vi "Modbus RT Driver VI.vi"(6 "Device Clock":string, 9 "Device Inputs FIFO":refnum<k33>, 10 "Device Outputs FIFO":refnum<k33>, 11 "Device Reference":T11 format="%.0x") -> ()   [LabVIEW 2014, in "Modbus Engine.lvlib"]
uses:
  Modbus Engine.lvlib
  <vilib>/NI Veristand/Custom Device API/Custom Device Item Ref.ctl
  XML Deserializer/XML VIs/API/Controls/Modbus_Items.ctl
  XML Deserializer/XML VIs/API/Controls/Modbus_Item_Type.ctl
  Shared/FIFO Indexes.ctl
  <vilib>/NI Veristand/Custom Device API/Custom Device Channel Type.ctl
  XML Deserializer/XML VIs/API/Controls/Modbus_General_Settings.ctl
  XML Deserializer/XML VIs/API/Controls/Modbus_Communication_Type.ctl
  XML Deserializer/XML VIs/API/Controls/Modbus_Type.ctl
  XML Deserializer/XML VIs/API/Controls/Modbus_Serial_Settings_Flow_Control.ctl
  XML Deserializer/XML VIs/API/Controls/Modbus_Serial_Settings_Parity.ctl
  XML Deserializer/XML VIs/API/Controls/Modbus_Serial_Settings_Serial_Type.ctl
  <vilib>/NI Veristand/Custom Device API/Message Response (String).ctl
  <vilib>/NI Veristand/Custom Device API/Message Response (Byte Array).ctl
  <vilib>/NI Veristand/Custom Device Tools/Custom Device Utility Library/RT Debug String Color Spec.ctl
  <vilib>/NI Veristand/Custom Device API/Get Item Property (Variant).vi
  Glyphs/Modbus Property Names.vi
  <vilib>/NI Veristand/Custom Device API/Custom Device API.lvlib
  <vilib>/NI Veristand/Custom Device Tools/Custom Device Utility Library/Custom Device Utility Library.lvlib
  Shared/Modbus Shared.lvlib
  <vilib>/NI_Real-Time Target Support.lvlib
panel:
  in  "Inputs RT-FIFO":dbl[](array[numeric])=[0.0, 0.0, 0.0, 0.0, 0.0, 0.0, 0.0, 0.0, 0.0, 0.0, 0.0, 0.0, 0.0, 0.0, 0.0, 0.0, 0.0, 0.0, 0.0, 0.0, 0.0, 0.0, 0.0, 0.0, 0.0, 0.0, 0.0, 0.0, 0.0, 0.0]
  out "Outputs RT-FIFO":dbl[](array[numeric])
  out "DEBUG error IO":errorcluster
  in  "DEBUG stop":bool
  out "DEBUG General Settings":T1 {"Communication_Type" items=["TCP", "Serial"]; "Modbus_Type" items=["Master", "Slave"]; "Serial Settings"."Serial_Settings_Flow_Control" items=["None", "XONXOFF", "RTSCTS", "XONXOFFANDRTSCTS", "DTRDSR", "XONXOFFANDDTRDSR"]; "Serial Settings"."Serial_Settings_Parity" items=["None", "Odd", "Even"]; "Serial Settings"."Serial_Settings_Serial_Type" items=["RTU", "ASCII"]}
  out "DEBUG RT-FIFOs Indexes":T7[](array[typedef])
  out "DEBUG Modbus Items":T9[](array[typedef])
  in  "Initialization Status Notifier":refnum<notifier>
  in  "Status Notifier":refnum<notifier>
  # "Custom Device Template\nv1.0"
  # "Use this template as a starting point for creating a custom device code module. The input controls shown here are specially named controls that the system will use to provide the device loop with data. The controls are not required for the device loop to run. For instance, if the device doesn't produce any output data, then you don't need the Device Outputs FIFO control. If you do use these controls, however, they need to have these exact names to be functional."
  # "The optional status notifier element is used to notify the RT engine of the last state of the custom device, and to indicate the device has completed execution. If this control is not used, a default No Error value is returned to the system when the device finishes execution.\n\nNote: This error state is not checked until the system shuts down. Use an output status channel to send more immediate status values to the system."
  # "This optional input can be used to send the VeriStand Engine the final status of the custom device initalization process. If this control exists on the custom device front panel, the VeriStand Engine will wait for a status update before starting up. If the custom device reports an error, that will abort the execution of the current configuration in the VeriStand Engine.\n\nThis control can be deleted if the custom device does not need to send the initialization status update."
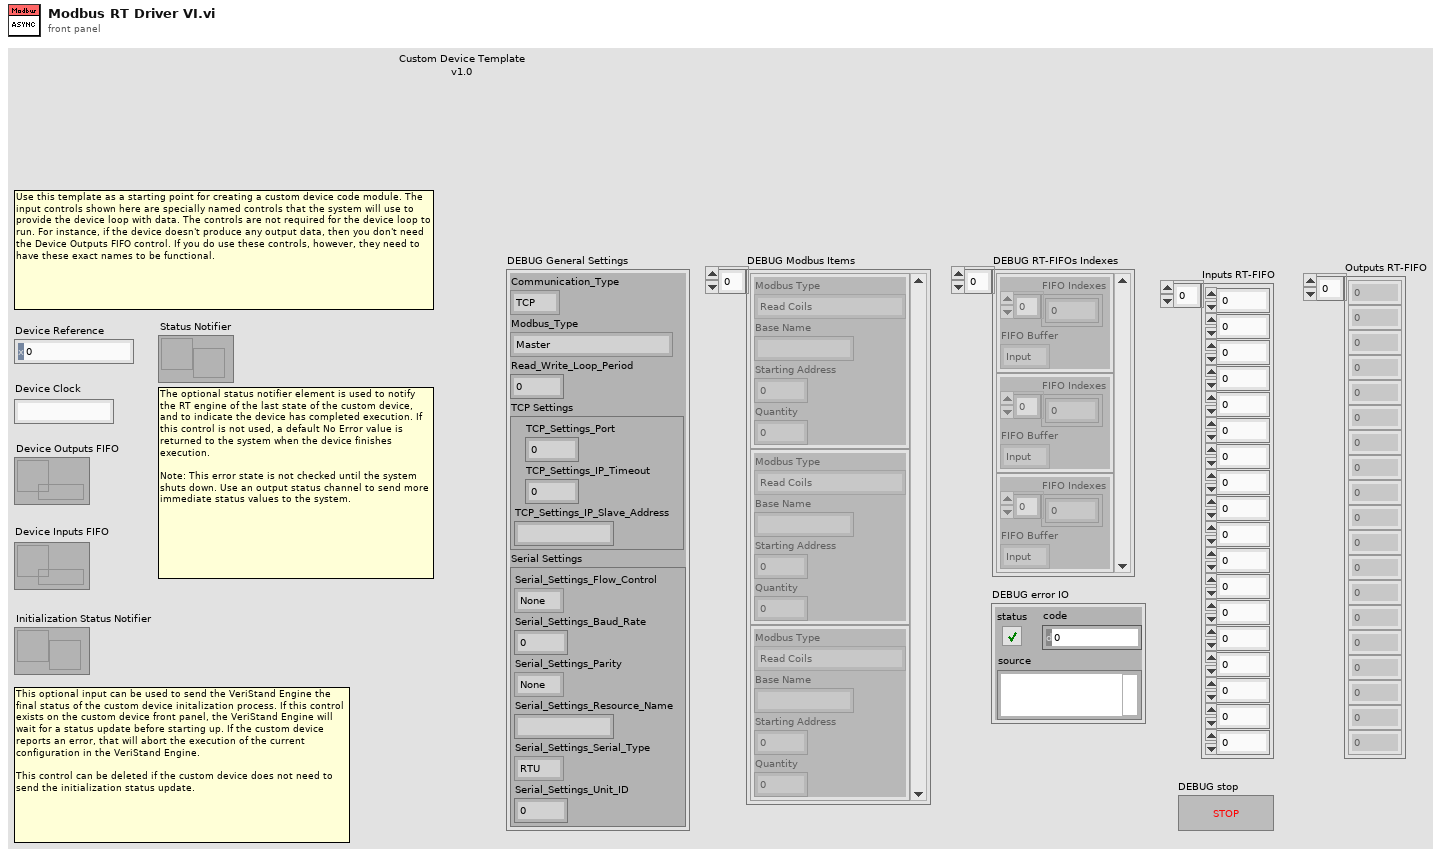
[diagram p1: front panel]
types:
  T1 = typedef "Modbus Shared.lvlib/Modbus_General_Settings.ctl" = cluster{"Communication_Type":T2, "Modbus_Type":T3, "Read_Write_Loop_Period":i64, "TCP Settings":cluster{"TCP_Settings_Port":u16, "TCP_Settings_IP_Timeout":u32, "TCP_Settings_IP_Slave_Address":string}, "Serial Settings":cluster{"Serial_Settings_Flow_Control":T4, "Serial_Settings_Baud_Rate":u32, "Serial_Settings_Parity":T5, "Serial_Settings_Resource_Name":string, "Serial_Settings_Serial_Type":T6, "Serial_Settings_Unit_ID":u8}}
  T2 = typedef "Modbus Shared.lvlib/Modbus_Communication_Type.ctl" = i32
  T3 = typedef "Modbus Shared.lvlib/Modbus_Type.ctl" = i32
  T4 = typedef "Modbus Shared.lvlib/Modbus_Serial_Settings_Flow_Control.ctl" = i32
  T5 = typedef "Modbus Shared.lvlib/Modbus_Serial_Settings_Parity.ctl" = i32
  T6 = typedef "Modbus Shared.lvlib/Modbus_Serial_Settings_Serial_Type.ctl" = i32
  T7 = typedef "Modbus Shared.lvlib/FIFO Indexes.ctl" = cluster{"FIFO Indexes":i32[], "FIFO Buffer":T8}
  T8 = typedef "Custom Device API.lvlib/Custom Device Channel Type.ctl" = enum16{"Input", "Output"}
  T9 = typedef "Modbus Shared.lvlib/Modbus_Items.ctl" = cluster{"Modbus Type":T10, "Base Name":string, "Starting Address":u16, "Quantity":u16}
  T10 = typedef "Modbus Shared.lvlib/Modbus_Item_Type.ctl" = enum16{"Read Coils", "Read Discrete Inputs", "Read Holding Registers", "Read Input Registers", "Write Multiple Coils", "Write Multiple Holding Registers", "Write Single Coil", "Write Single Holding Register", "Write Multiple Discrete Inputs", "Write Multiple Input Registers"}
  T11 = typedef "Custom Device API.lvlib/Custom Device Item Ref.ctl" = u64
  T12 = typedef "Custom Device API.lvlib/Custom Device Item Info.ctl" = cluster{"Name":string, "Is Channel":bool, "GUID":string, "Is Waveform":bool}
  T13 = typedef "Custom Device API.lvlib/Custom Device Engine Event Ref.ctl" = refnum<event-registration>
  T14 = cluster{"TCP_Settings_Port":u16, "TCP_Settings_IP_Timeout":u32, "TCP_Settings_IP_Slave_Address":string}
  T15 = cluster{"Serial_Settings_Flow_Control":T4, "Serial_Settings_Baud_Rate":u32, "Serial_Settings_Parity":T5, "Serial_Settings_Resource_Name":string, "Serial_Settings_Serial_Type":T6, "Serial_Settings_Unit_ID":i8}
  T16 = typedef "Custom Device API.lvlib/Message Response (String).ctl" = cluster{"Response":string, "Error":errorcluster}
  T17 = typedef "Custom Device API.lvlib/Message Response (Byte Array).ctl" = cluster{"Response":u8[], "Error":errorcluster}
  T18 = typedef "Custom Device Utility Library.lvlib/RT Debug String Color Spec.ctl" = u16
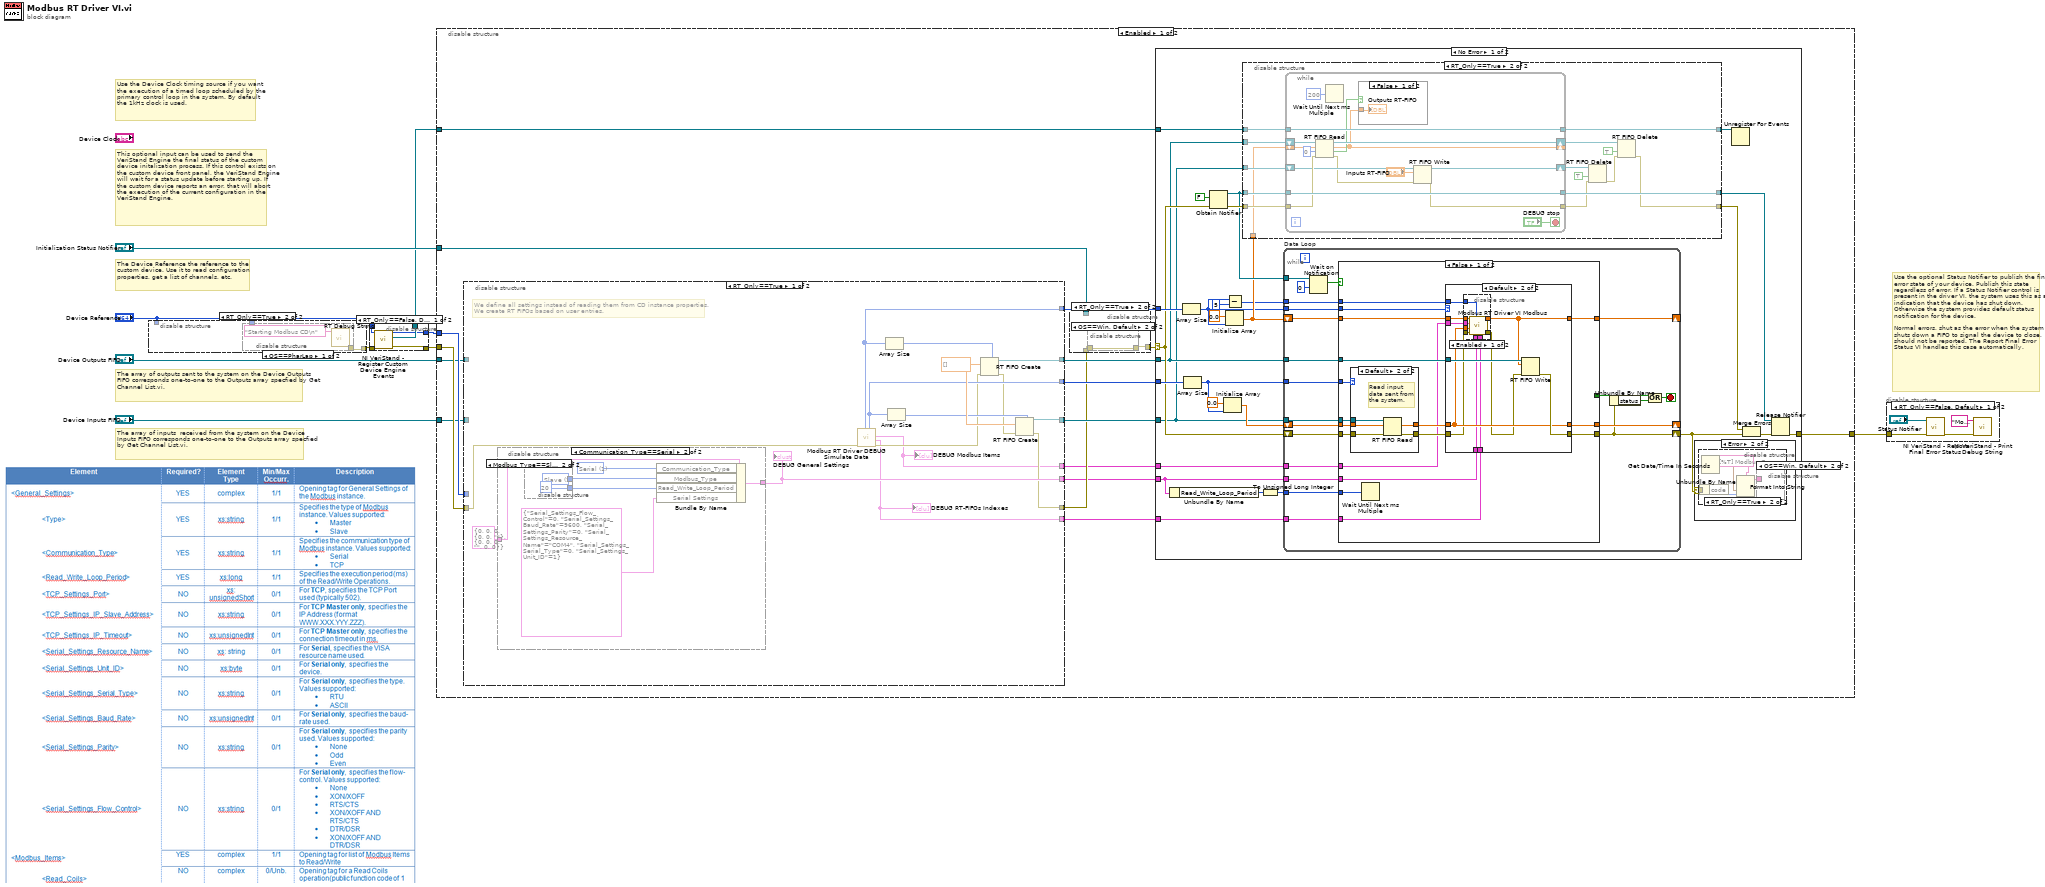
[diagram p0: block diagram]
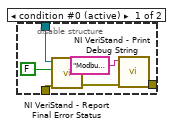
[diagram p2: hidden frame]
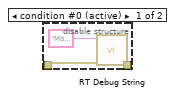
[diagram p3: hidden frame]
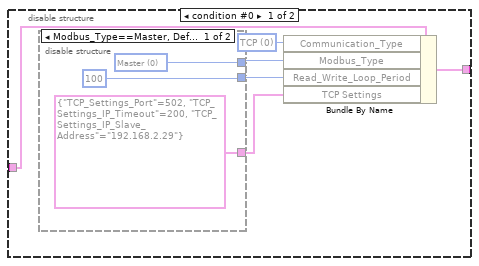
[diagram p4: hidden frame]
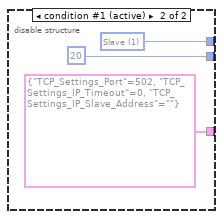
[diagram p5: hidden frame]
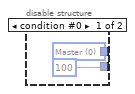
[diagram p6: hidden frame]
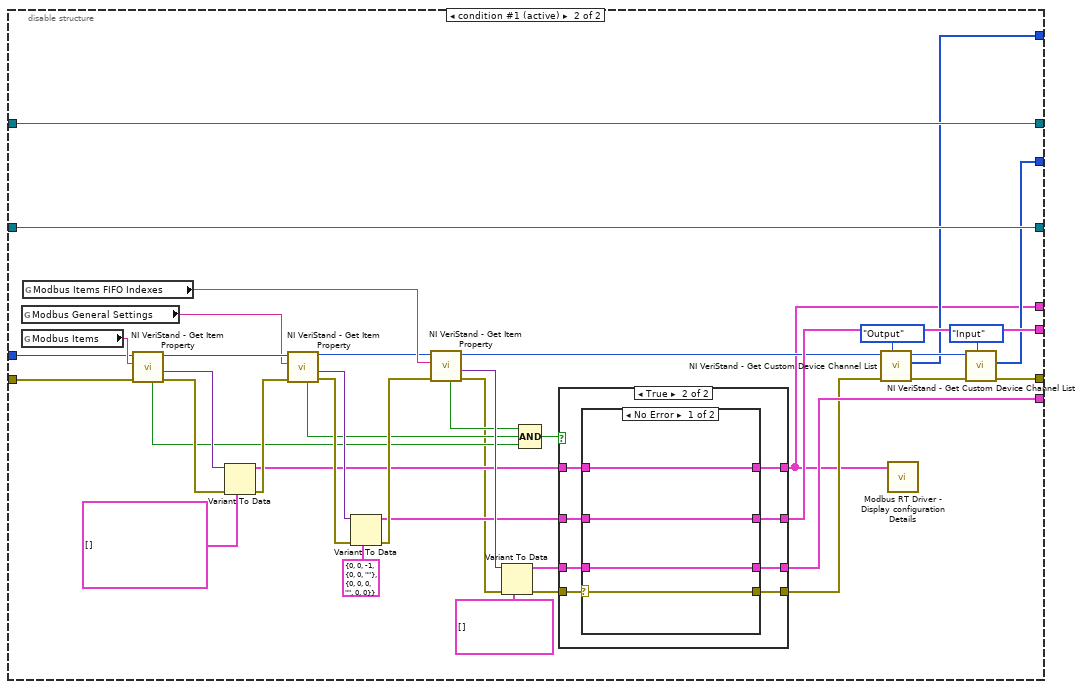
[diagram p7: hidden frame]
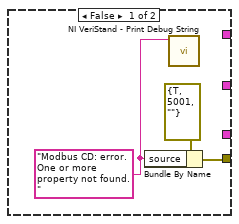
[diagram p8: hidden frame]
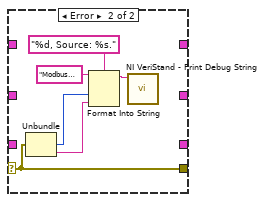
[diagram p9: hidden frame]
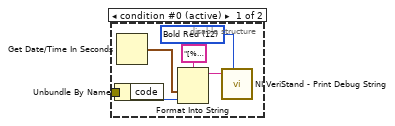
[diagram p11: hidden frame]
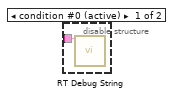
[diagram p12: hidden frame]
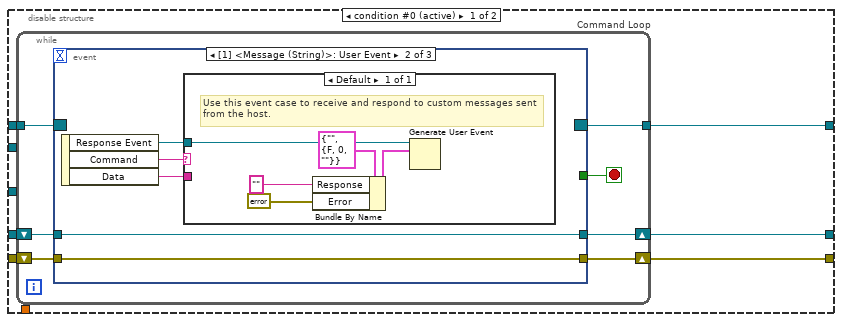
[diagram p13: hidden frame]
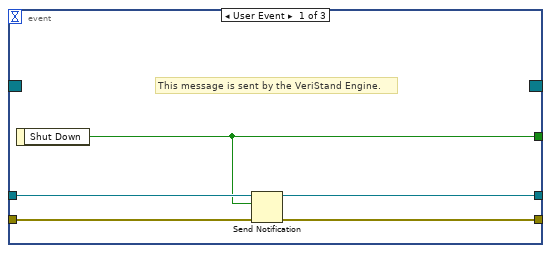
[diagram p14: hidden frame]
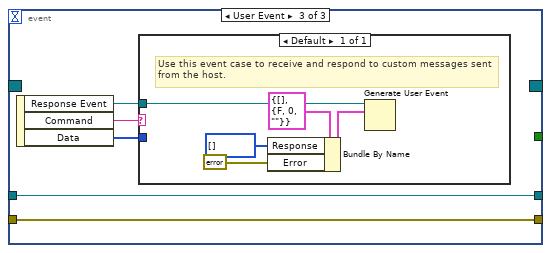
[diagram p15: hidden frame]
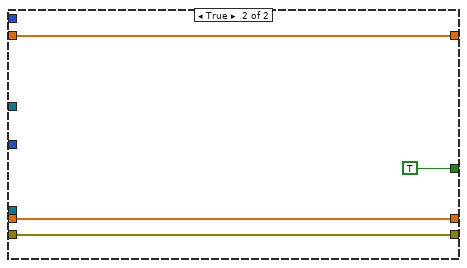
[diagram p20: hidden frame]
diagram:
  # "This optional input can be used to send the VeriStand Engine the final status of the custom device initalization process. If this control exists on the custom device front panel, the VeriStand Engine will wait for a status update before starting up. If the custom device reports an error, that will abort the execution of the current configuration in the VeriStand Engine."
  # "The array of inputs  received from the system on the Device Inputs FIFO corresponds one-to-one to the Outputs array specfied by Get Channel List.vi."
  # "Use the optional Status Notifier to publish the final error state of your device. Publish this state regardless of error. If a Status Notifier control is present in the driver VI, the system uses this as an indication that the device has shut down. Otherwise the system provides default status notification for the device.\n\nNormal errors, shut as the error when the system shuts down a FIFO to signal the device to close, should not be reported. The Report Final Error Status VI handles this case automatically."
  # "The array of outputs sent to the system on the Device Outputs FIFO corresponds one-to-one to the Outputs array specfied by Get Channel List.vi."
  # "The Device Reference the reference to the custom device. Use it to read configuration properties, get a list of channels, etc."
  # "Use the Device Clock timing source if you want the execution of a timed loop scheduled by the primary control loop in the system. By default the 1kHz clock is used."
  n1 = disable-structure shown="RT_Only==True" {
    disable-tunnel: [w25 w26] -> w6
    disable-tunnel: "Device Reference" -> [w17 _]
    disable-tunnel: "Device Reference" -> [w15 _]
    frame condition #0 (active) {
      n2 = call <vilib>:"NI VeriStand - Get Custom Device Version.vi"("Device Ref in"=w17) -> ("error out"=w13:errorcluster, "Value"=w11:string)  [unwired: 8 in, 1 out]
      n3 = Concatenate Strings("Modbus CD: Version " ("Message"), w11, "\r") -> (w14:string)
      n4 = call <vilib>:"NI VeriStand - Print Debug String.vi"("error in (no error)"=w13, "Message"=w14) -> ("error out"=w16:errorcluster)  [unwired: 9 in]
      n5 = call <vilib>:"NI VeriStand - Get Item Data.vi"("error in (no error)"=w16, "Item Ref in"=w15) -> ("error out"=w24:errorcluster, "Item Info"=w21:T12)  [unwired: 6 in, 2 out]
      n6 = Unbundle By Name(w21) -> ("Name"=w20:string)
      n7 = Format Into String(format string="%s%s", initial string="Modbus CD instance \"" ("Message"), w20, "\": code initialization.\n" ("Message")) -> (resulting string=w23:string)  [unwired: 1 in, 1 out]
      n8 = call <vilib>:"NI VeriStand - Print Debug String.vi"("error in (no error)"=w24, "Message"=w23) -> ("error out"=w25:errorcluster)  [unwired: 9 in]
    }
    frame condition #1 {
      n9 = disable-structure shown="OS==PharLap" {
        disable-tunnel: [w28 _] -> w26
        frame condition #0 (active) {
          n10 = call <vilib>:"RT Debug String.vi"("String to write"="Starting Modbus CD\n") -> ("error out"=w28:errorcluster)  [unwired: 10 in]
        }
        frame condition #1 {
        }
      }
    }
  }
  n11 = disable-structure shown="RT_Only==False, Default" {
    disable-tunnel: [w33 _] -> w8
    disable-tunnel: "Device Reference" -> [w32 _]
    disable-tunnel: w6 -> [w31 w34]
    disable-tunnel: [w30 w34] -> w5
    disable-tunnel: [w29 _] -> w4
    frame condition #0 (active) {
      n12 = call <vilib>:"NI VeriStand - Register Custom Device Engine Events.vi"("error in (no error)"=w31, "Device Ref in"=w32) -> ("error out"=w30:errorcluster, "Custom Device Engine Event Ref"=w33:T13, "Device Ref out"=w29:T11)  [unwired: 7 in]
    }
    frame condition #1 {
    }
  }
  n13 = disable-structure shown="Enabled" {
    disable-tunnel: "Initialization Status Notifier" -> [w50 _]
    disable-tunnel: w8 -> [w49 _]
    disable-tunnel: [w48 w347] -> w7
    disable-tunnel: w5 -> [w46 w347]
    disable-tunnel: w4 -> [w45 _]
    disable-tunnel: "Device Inputs FIFO" -> [w44 _]
    disable-tunnel: "Device Outputs FIFO" -> [w42 _]
    frame Enabled {
      n14 = disable-structure shown="RT_Only==True" {
        disable-tunnel: [w64 w100] -> w35
        disable-tunnel: [w66 w101] -> w38
        disable-tunnel: [w76 w115] -> w37
        disable-tunnel: [w63 w114] -> w36
        disable-tunnel: w46 -> [w68 w113]
        disable-tunnel: w45 -> [_ w112]
        disable-tunnel: w44 -> [_ w111]
        disable-tunnel: [w74 w111] -> w43
        disable-tunnel: w42 -> [_ w110]
        disable-tunnel: [w75 w110] -> w41
        disable-tunnel: [w72 w105] -> w40
        disable-tunnel: [w70 w104] -> w39
        frame condition #0 {
          w73 = dbl[] []
          # "We define all settings instead of reading them from CD instance properties.\nWe create RT FIFOs based on user entries."
          n15 = disable-structure shown="Communication_Type==Serial" {
            disable-tunnel: T1 {"Communication_Type"=0, "Modbus_Type"=0, "Read_Write_Loop_Period"=0, "TCP Settings"={"TCP_Settings_Port"=0, "TCP_Settings_IP_Timeout"=0, "TCP_Settings_IP_Slave_Address"=""}, "Serial Settings"={"Serial_Settings_Flow_Control"=0, "Serial_Settings_Baud_Rate"=0, "Serial_Settings_Parity"=0, "Serial_Settings_Resource_Name"="", "Serial_Settings_Serial_Type"=0, "Serial_Settings_Unit_ID"=0}} ("DEBUG General Settings") -> [w83 w95]
            disable-tunnel: [w81 w93] -> w76
            frame condition #0 {
              w82 = T2 0 items=["TCP", "Serial"] ("Communication_Type")
              n16 = disable-structure shown="Modbus_Type==Master, Default" {
                disable-tunnel: [w86 w89] -> w79
                disable-tunnel: [i64 100 ("Read_Write_Loop_Period") i64 20 ("Read_Write_Loop_Period")] -> w80
                disable-tunnel: [T14 {"TCP_Settings_Port"=502, "TCP_Settings_IP_Timeout"=200, "TCP_Settings_IP_Slave_Address"="192.168.2.29"} ("TCP Settings") T14 {"TCP_Settings_Port"=502, "TCP_Settings_IP_Timeout"=0, "TCP_Settings_IP_Slave_Address"=""} ("TCP Settings")] -> w78
                frame condition #0 {
                  w86 = T3 0 items=["Master", "Slave"] ("Modbus_Type")
                }
                frame condition #1 (active) {
                  w89 = T3 1 items=["Master", "Slave"] ("Modbus_Type")
                }
              }
              n17 = Bundle By Name(cluster=w83, "Communication_Type"=w82, "Modbus_Type"=w79, "Read_Write_Loop_Period"=w80, "TCP Settings"=w78) -> (w81:T1)
            }
            frame condition #1 (active) {
              w94 = T2 1 items=["TCP", "Serial"] ("Communication_Type")
              n18 = disable-structure shown="Modbus_Type==Slave" {
                disable-tunnel: [w97 w99] -> w91
                disable-tunnel: [i64 100 ("Read_Write_Loop_Period") i64 20 ("Read_Write_Loop_Period")] -> w92
                frame condition #0 {
                  w97 = T3 0 items=["Master", "Slave"] ("Modbus_Type")
                }
                frame condition #1 (active) {
                  w99 = T3 1 items=["Master", "Slave"] ("Modbus_Type")
                }
              }
              n19 = Bundle By Name(cluster=w95, "Communication_Type"=w94, "Modbus_Type"=w91, "Read_Write_Loop_Period"=w92, "Serial Settings"=T15 {"Serial_Settings_Flow_Control"=0, "Serial_Settings_Baud_Rate"=9600, "Serial_Settings_Parity"=0, "Serial_Settings_Resource_Name"="COM4", "Serial_Settings_Serial_Type"=0, "Serial_Settings_Unit_ID"=1}) -> (w93:T1)
            }
          }
          "DEBUG General Settings" <- w76
          n20 = call "Modbus RT Driver DEBUG Simulate Data.vi"("error in (no error)"=w68) -> ("error out"=w65:errorcluster, "DEBUG RT-FIFOs Indexes"=w63:T7[], "DEBUG Modbus Items"=w64:T9[], "Input Specified Channel Ref List"=w70:T11[], "Output Specified Channel Ref List"=w72:T11[])  [unwired: 6 in]
          "DEBUG Modbus Items" <- w64
          "DEBUG RT-FIFOs Indexes" <- w63
          n21 = Array Size(array=w72) -> (size(s)=w71:i32)
          n22 = Array Size(array=w70) -> (size(s)=w69:i32)
          n23 = RT FIFO Create(1:w73, 3:w65, 6:w71) -> (8:w75:refnum<k33>, 11:w67:errorcluster)  [unwired: 5 in, 1 out]
          n24 = RT FIFO Create(1:w73, 3:w67, 6:w69) -> (8:w74:refnum<k33>, 11:w66:errorcluster)  [unwired: 5 in, 1 out]
        }
        frame condition #1 (active) {
          n25 = global read "Modbus Property Names.vi" "Modbus General Settings"() -> (w136:string)
          n26 = global read "Modbus Property Names.vi" "Modbus Items"() -> (w135:string)
          n27 = global read "Modbus Property Names.vi" "Modbus Items FIFO Indexes"() -> (w139:string)
          n28 = call-poly <vilib>:"NI VeriStand - Get Item Property.vi"("error in (no error)"=w113, "Property Name"=w135, "Item Ref in"=w112) -> ("error out"=w128:errorcluster, "Value"=w134:variant, "Item Ref out"=w138:T11, "Found?"=w123:bool)  [unwired: 5 in]
          n29 = Variant To Data(error in=w128, type=T9[] [], Variant=w134) -> (data=w118:T9[], error out=w133:errorcluster)
          n30 = call-poly <vilib>:"NI VeriStand - Get Item Property.vi"("error in (no error)"=w133, "Property Name"=w136, "Item Ref in"=w138) -> ("error out"=w132:errorcluster, "Value"=w131:variant, "Item Ref out"=w137:T11, "Found?"=w124:bool)  [unwired: 5 in]
          n31 = Variant To Data(error in=w132, type=T1 {"Communication_Type"=0, "Modbus_Type"=0, "Read_Write_Loop_Period"=-1, "TCP Settings"={"TCP_Settings_Port"=0, "TCP_Settings_IP_Timeout"=0, "TCP_Settings_IP_Slave_Address"=""}, "Serial Settings"={"Serial_Settings_Flow_Control"=0, "Serial_Settings_Baud_Rate"=0, "Serial_Settings_Parity"=0, "Serial_Settings_Resource_Name"="", "Serial_Settings_Serial_Type"=0, "Serial_Settings_Unit_ID"=0}} ("General Settings"), Variant=w131) -> (data=w119:T1, error out=w127:errorcluster)
          n32 = call-poly <vilib>:"NI VeriStand - Get Item Property.vi"("error in (no error)"=w127, "Property Name"=w139, "Item Ref in"=w137) -> ("error out"=w116:errorcluster, "Value"=w130:variant, "Item Ref out"=w103:T11, "Found?"=w125:bool)  [unwired: 5 in]
          n33 = Variant To Data(error in=w116, type=T7[] [], Variant=w130) -> (data=w120:T7[], error out=w117:errorcluster)
          n34 = Compound Arithmetic op=AND(w125, w124, w123) -> (w122:bool)
          n35 = case shown="True" w122 {
            tunnel: w120 -> [_ w147]
            tunnel: w119 -> [_ w148]
            tunnel: w118 -> [_ w149]
            tunnel: w117 -> [_ w150]
            tunnel: [_ w146] -> w100
            tunnel: [_ w145] -> w115
            tunnel: [_ w144] -> w114
            tunnel: [w141 w143] -> w102
            frame False {
              w140 = "Modbus CD: error. One or more property not found." ("source")
              n36 = Bundle By Name(cluster=errorcluster {"status"=TRUE, "code"=5001, "source"=""} ("error IO"), "source"=w140) -> (w141:errorcluster)
              n37 = call <vilib>:"NI VeriStand - Print Debug String.vi"("Message"=w140) -> ()  [unwired: 10 in, 1 out]
            }
            frame True {
              n38 = case shown="No Error" w150 {
                selector: w150 -> [w151 w158]
                tunnel: w149 -> [w154 _]
                tunnel: w148 -> [w153 _]
                tunnel: w147 -> [w152 _]
                tunnel: [w154 _] -> w146
                tunnel: [w153 _] -> w145
                tunnel: [w152 _] -> w144
                tunnel: [w151 w158] -> w143
                frame No Error {
                }
                frame Error {
                  n39 = Unbundle(w158) -> ("code"=w157:i32, "source"=w156:string)  [unwired: 1 out]
                  n40 = Format Into String(format string="%d, Source: %s.", initial string="Modbus CD: error. Code: " ("source"), w157, w156) -> (resulting string=w159:string)  [unwired: 1 in, 1 out]
                  n41 = call <vilib>:"NI VeriStand - Print Debug String.vi"("Message"=w159) -> ()  [unwired: 10 in, 1 out]
                }
              }
            }
          }
          n42 = call <vilib>:"NI VeriStand - Get Custom Device Channel List.vi"("Channel Type"=Custom_Device_Channel_Type."Output", "error in (no error)"=w102, "Device Ref in"=w103) -> ("error out"=w108:errorcluster, "Specified Channel Ref List"=w105:T11[], "Device Ref out"=w107:T11)  [unwired: 6 out]
          n43 = call "Modbus RT Driver - Display configuration Details.vi"("Array"=w100) -> ()  [unwired: 11 in]
          n44 = call <vilib>:"NI VeriStand - Get Custom Device Channel List.vi"("Channel Type"=Custom_Device_Channel_Type."Input", "error in (no error)"=w108, "Device Ref in"=w107) -> ("error out"=w101:errorcluster, "Specified Channel Ref List"=w104:T11[])  [unwired: 7 out]
        }
      }
      n45 = disable-structure shown="RT_Only==True" {
        disable-tunnel: w50 -> [w56 _]
        disable-tunnel: [w54 w58] -> w47
        disable-tunnel: w38 -> [w52 w57]
        frame condition #0 (active) {
          n46 = call <vilib>:"NI VeriStand - Report Final Error Status.vi"("error in (no error)"=w52, "Filter FIFO & Shutdown Errors (T)"=FALSE ("Filter FIFO Errors (T)"), "Status Notifier"=w56) -> ("error out"=w53:errorcluster)  [unwired: 8 out]
          n47 = call <vilib>:"NI VeriStand - Print Debug String.vi"("error in (no error)"=w53, "Message"="Modbus CD: initialization completed.\n") -> ("error out"=w54:errorcluster)  [unwired: 9 in]
        }
        frame condition #1 {
          n48 = disable-structure shown="OS==Win, Default" {
            disable-tunnel: [w61 w62] -> w58
            disable-tunnel: w57 -> [w60 w62]
            frame condition #0 (active) {
              n49 = call <vilib>:"RT Debug String.vi"("error in (no error)"=w60, "String to write"="Modbus CD Initialized\n") -> ("error out"=w61:errorcluster)  [unwired: 9 in]
            }
            frame condition #1 {
            }
          }
        }
      }
      n50 = case shown="No Error" w47 {
        selector: w47 -> [w175 w346]
        tunnel: w41 -> [w172 _]
        tunnel: w43 -> [w171 _]
        tunnel: w39 -> [w184 _]
        tunnel: w40 -> [w183 _]
        tunnel: w49 -> [w181 _]
        tunnel: [w179 w346] -> w48
        tunnel: w37 -> [w169 _]
        tunnel: w36 -> [w170 _]
        tunnel: w35 -> [w166 _]
        frame No Error {
          n51 = Unbundle By Name(w169) -> ("Read_Write_Loop_Period"=w168:i64)
          n52 = Array Size(array=w183) -> (size(s)=w164:i32)
          n53 = Array Size(array=w184) -> (size(s)=w182:i32)
          n54 = Obtain Notifier(notification data type=FALSE ("Shut Down"), error in (no error)=w175) -> (notifier out=w177:refnum<notifier>, error out=w188:errorcluster)  [unwired: 2 in, 1 out]
          n55 = Initialize Array(0.0 ("element"), w182) -> (w185:dbl[])
          n56 = Initialize Array(0.0 ("element"), w164) -> (w165:dbl[])
          n57 = Subtract(x=w164, y=5) -> (x-y=w162:i32)
          n58 = disable-structure shown="RT_Only==True" {
            disable-tunnel: w188 -> [w207 w254]
            disable-tunnel: w181 -> [w206 w251]
            disable-tunnel: [w205 w250] -> w178
            disable-tunnel: w177 -> [w204 w253]
            disable-tunnel: [w203 w252] -> w176
            disable-tunnel: [w202 w243] -> w173
            disable-tunnel: w172 -> [_ w249]
            disable-tunnel: w171 -> [_ w248]
            disable-tunnel: w165 -> [_ w240]
            frame condition #0 (active) {
              n59 = while "Command Loop" {
                tunnel: w206 -> [w214]
                tunnel: [w213] -> w205
                shift-right: [w210] -> w203
                shift-left: w204 -> [w211]
                shift-right: [w208] -> w202
                shift-left: w207 -> [w209]
                stop <- w212 stop-if-true
                n60 = event shown="[1] <Message (String)>: User Event" {
                  selector: w214 -> [_ _ _]
                  dyn-events: [_ _ _] -> w213
                  timeout: _ -> [_ _ _]
                  tunnel: [w217 _ _] -> w212
                  tunnel: w211 -> [w218 w222 w232]
                  tunnel: [w219 w222 w232] -> w210
                  tunnel: w209 -> [w216 w220 w230]
                  tunnel: [w215 w220 w230] -> w208
                  event User Event {
                    # "This message is sent by the VeriStand Engine."
                    n61 = event-data() -> ("Shut Down"=w217:bool)  [unwired: 1 in]
                    n62 = Send Notification(notification=w217, notifier=w218, error in (no error)=w216) -> (notifier out=w219:refnum<notifier>, error out=w215:errorcluster)
                  }
                  event User Event {
                    n63 = event-data() -> ("Response Event"=w221:refnum<user-event>, "Command"=w224:string, "Data"=w223:string)  [unwired: 1 in]
                    n64 = case shown="Default" w224 {
                      tunnel: w223 -> [_]
                      tunnel: w221 -> [w229]
                      frame Default {
                        # "Use this event case to receive and respond to custom messages sent from the host."
                        n65 = Bundle By Name(cluster=T16 {"Response"="", "Error"={"status"=FALSE, "code"=0, "source"=""}} ("event data"), "Response"="", "Error"=errorcluster {"status"=FALSE, "code"=0, "source"=""}) -> (w227:T16)
                        n66 = Generate User Event(user event=w229, event data cluster=w227) -> ()  [unwired: 2 in, 2 out]
                      }
                    }
                  }
                  event User Event {
                    n67 = event-data() -> ("Response Event"=w231:refnum<user-event>, "Command"=w234:string, "Data"=w233:u8[])  [unwired: 1 in]
                    n68 = case shown="Default" w234 {
                      tunnel: w233 -> [_]
                      tunnel: w231 -> [w239]
                      frame Default {
                        # "Use this event case to receive and respond to custom messages sent from the host."
                        n69 = Bundle By Name(cluster=T17 {"Response"=[], "Error"={"status"=FALSE, "code"=0, "source"=""}} ("event data"), "Response"=u8[] [], "Error"=errorcluster {"status"=FALSE, "code"=0, "source"=""}) -> (w236:T17)
                        n70 = Generate User Event(user event=w239, event data cluster=w236) -> ()  [unwired: 2 in, 2 out]
                      }
                    }
                  }
                }
              }
            }
            frame condition #1 {
              n71 = while {
                tunnel: w254 -> [w264]
                tunnel: [w256] -> w247
                tunnel: w253 -> [w270]
                tunnel: [w270] -> w252
                tunnel: w251 -> [w269]
                tunnel: [w269] -> w250
                shift-right: [w260] -> _
                shift-left: w240 -> [w263]
                shift-right: [w265] -> w245
                shift-left: w249 -> [w266]
                shift-right: [w258] -> w246
                shift-left: w248 -> [w259]
                stop <- "DEBUG stop" stop-if-true
                n72 = RT FIFO Read(0:w266, 1:w263, 2:0 ("timeout in ms (0)"), 3:w264) -> (8:w265:refnum<k33>, 9:w260:dbl[], 10:w261:bool, 11:w257:errorcluster)  [unwired: 1 out]
                n73 = Wait Until Next ms Multiple(millisecond multiple=u32 200) -> ()  [unwired: 1 out]
                n74 = case shown="False" w261 {
                  tunnel: w260 -> [w271 _]
                  frame False {
                    "Outputs RT-FIFO" <- w271
                  }
                  frame True {
                  }
                }
                n75 = RT FIFO Write(0:w259, 1:"Inputs RT-FIFO", 3:w257) -> (8:w258:refnum<k33>, 11:w256:errorcluster)  [unwired: 2 in, 2 out]
              }
              n76 = RT FIFO Delete(0:w246, 2:TRUE ("force destroy? (F)"), 3:w247) -> (11:w244:errorcluster)
              n77 = RT FIFO Delete(0:w245, 2:TRUE ("force destroy? (F)"), 3:w244) -> (11:w243:errorcluster)
            }
          }
          n78 = To Unsigned Long Integer(number=w168) -> (unsigned 32bit integer=w167:u32)
          n79 = while "Data Loop" {
            shift-right: [w290] -> _
            shift-left: w185 -> [w291]
            shift-right: [w282] -> w161
            shift-left: w175 -> [w292]
            shift-right: [w288] -> _
            shift-left: w165 -> [w289]
            tunnel: w164 -> [w285]
            tunnel: w172 -> [w287]
            tunnel: w171 -> [w286]
            tunnel: w182 -> [w284]
            tunnel: w177 -> [w281]
            tunnel: w169 -> [w276]
            tunnel: w170 -> [w275]
            tunnel: w167 -> [w274]
            tunnel: w166 -> [w273]
            tunnel: w162 -> [w272]
            stop <- w277 stop-if-true
            n80 = Wait on Notification(notifier=w281, timeout in ms (-1)=0) -> (notification=w280:bool)  [unwired: 2 in, 3 out]
            n81 = case shown="False" w280 {
              tunnel: w292 -> [w309 w344]
              tunnel: w291 -> [w308 w345]
              tunnel: [w307 w345] -> w290
              tunnel: w289 -> [w306 w343]
              tunnel: [w305 w343] -> w288
              tunnel: w287 -> [w304 _]
              tunnel: w286 -> [w303 _]
              tunnel: w285 -> [w302 _]
              tunnel: w284 -> [w301 _]
              tunnel: [w298 w344] -> w282
              tunnel: [_ TRUE] -> w278
              tunnel: w276 -> [w295 _]
              tunnel: w275 -> [w294 _]
              tunnel: w274 -> [w297 _]
              tunnel: w273 -> [w296 _]
              tunnel: w272 -> [w293 _]
              frame False {
                n82 = case shown="Default" w301 {
                  tunnel: w303 -> [_ w341]
                  tunnel: w308 -> [w336 w340]
                  tunnel: [w336 w339] -> w300
                  tunnel: [w335 w338] -> w299
                  tunnel: w309 -> [w335 w337]
                  frame 0 {
                  }
                  frame Default {
                    # "Read input data sent from the system."
                    n83 = RT FIFO Read(0:w341, 1:w340, 3:w337) -> (9:w339:dbl[], 11:w338:errorcluster)  [unwired: 4 out]
                  }
                }
                n84 = Wait Until Next ms Multiple(millisecond multiple=w297) -> ()  [unwired: 1 out]
                n85 = case shown="Default" w302 {
                  tunnel: w304 -> [_ w323]
                  tunnel: w306 -> [w312 w317]
                  tunnel: w300 -> [w311 w320]
                  tunnel: w299 -> [w310 w319]
                  tunnel: [w310 w322] -> w298
                  tunnel: [w312 w321] -> w305
                  tunnel: [w311 w320] -> w307
                  tunnel: w296 -> [_ w316]
                  tunnel: w295 -> [_ w315]
                  tunnel: w294 -> [_ w314]
                  tunnel: w293 -> [_ w313]
                  frame 0 {
                  }
                  frame Default {
                    n86 = disable-structure shown="Enabled" {
                      disable-tunnel: [w332 w334] -> w321
                      disable-tunnel: w320 -> [w331 _]
                      disable-tunnel: w319 -> [w330 w333]
                      disable-tunnel: [w329 w333] -> w318
                      disable-tunnel: w317 -> [w328 w334]
                      disable-tunnel: w316 -> [w327 _]
                      disable-tunnel: w315 -> [w326 _]
                      disable-tunnel: w314 -> [w325 _]
                      disable-tunnel: w313 -> [w324 _]
                      frame Enabled {
                        n87 = call "Modbus RT Driver VI Modbus.vi"("DEBUG RT-FIFOs Indexes"=w325, "DEBUG General Settings"=w326, "First FIFO Index of Status Channels"=w324, "error in (no error)"=w330, "Inputs In"=w331, "DEBUG Modbus Items"=w327, "Outputs In"=w328) -> ("error out"=w329:errorcluster, "Outputs Out"=w332:dbl[])  [unwired: 3 in]
                      }
                      frame Disabled {
                      }
                    }
                    n88 = RT FIFO Write(0:w323, 1:w321, 3:w318) -> (11:w322:errorcluster)  [unwired: 1 in, 4 out]
                  }
                }
              }
              frame True {
              }
            }
            n89 = Unbundle By Name(w282) -> ("status"=w279:bool)
            n90 = Compound Arithmetic op=OR(w278, w279) -> (w277:bool)
          }
          n91 = case shown="Error" w161 {
            selector: w161 -> [_ w189]
            frame No Error {
            }
            frame Error {
              n92 = disable-structure shown="RT_Only==True" {
                disable-tunnel: w189 -> [w195 w200]
                frame condition #0 (active) {
                  w190 = T18 12 items=["Plain White"=7, "Bold White"=15, "Bold Blue"=9, "Bold Green"=10, "Bold Red"=12] ("Attribute")
                  n93 = Unbundle By Name(w195) -> ("code"=w194:i32)
                  n94 = Get Date/Time In Seconds() -> (seconds since 1Jan1904=w192:timestamp)
                  n95 = Format Into String(format string="[%T] Modbus CD: Main VI: Error: %d\n", w192, w194) -> (resulting string=w193:string)  [unwired: 2 in, 1 out]
                  n96 = call <vilib>:"NI VeriStand - Print Debug String.vi"("Attribute"=w190, "Message"=w193) -> ()  [unwired: 9 in, 1 out]
                }
                frame condition #1 {
                  n97 = Unbundle By Name(w200) -> ("code"=w199:i32)
                  n98 = Get Date/Time In Seconds() -> (seconds since 1Jan1904=w198:timestamp)
                  n99 = Format Into String(format string="[%T] Modbus CD: Main VI: Error: %d\n", w198, w199) -> (resulting string=w196:string)  [unwired: 2 in, 1 out]
                  n100 = disable-structure shown="OS==Win, Default" {
                    disable-tunnel: w196 -> [w201 _]
                    frame condition #0 (active) {
                      n101 = call <vilib>:"RT Debug String.vi"("String to write"=w201) -> ()  [unwired: 10 in, 1 out]
                    }
                    frame condition #1 {
                    }
                  }
                }
              }
            }
          }
          n102 = Unregister For Events(event registration refnum=w178) -> ()  [unwired: 1 in, 1 out]
          n103 = Merge Errors(w173, w161) -> (w174:errorcluster)
          n104 = Release Notifier(notifier=w176, error in (no error)=w174) -> (error out=w179:errorcluster)  [unwired: 1 in, 2 out]
        }
        frame Error {
        }
      }
    }
    frame Disabled {
    }
  }
  n105 = disable-structure shown="RT_Only==False, Default" {
    disable-tunnel: w7 -> [w350 w352]
    frame condition #0 (active) {
      n106 = call <vilib>:"NI VeriStand - Report Final Error Status.vi"("error in (no error)"=w350, "Status Notifier"="Status Notifier") -> ("error out"=w349:errorcluster)  [unwired: 1 in, 8 out]
      n107 = call <vilib>:"NI VeriStand - Print Debug String.vi"("error in (no error)"=w349, "Message"="Modbus CD: code completed.\n") -> ()  [unwired: 9 in, 1 out]
    }
    frame condition #1 {
      "DEBUG error IO" <- w352
    }
  }
